vi "Event-Driven State Machine (Execution Log).vi"() -> ()   [LabVIEW 2020]
uses:
  support/States.ctl
  support/State Machine Data.ctl
  <vilib>/DAQmx/read.llb/DAQmx Read (Analog 2D DBL NChan NSamp).vi
  <vilib>/DAQmx/write.llb/DAQmx Write (Analog DBL 1Chan 1Samp).vi
  <vilib>/DAQmx/create/channels.llb/DAQmx Create Channel (AI-Voltage-Basic).vi
  <vilib>/DAQmx/configure/timing.llb/DAQmx Timing (Sample Clock).vi
  <vilib>/DAQmx/miscellaneous.llb/DAQmx Fill In Error Info.vi
  <vilib>/Utility/file.llb/Write Delimited Spreadsheet (DBL).vi
  <vilib>/DAQmx/create/channels.llb/DAQmx Create Channel (AO-Voltage-Basic).vi
panel:
  out "RMS Results Per Channel":dbl[](array[numeric])
  in  "AO Voltage Channel":tag="PCI-6221/ao1"
  in  "Generate Stimulus":bool
  out "Threshold exceeded?":bool
  in  "Acquire":bool
  in  "Samples per channel":i32=100
  in  "Sample Rate (Hz)":dbl=1000.0
  in  "AI Voltage Channel":tag="PCI-6221/ai0, PCI-6221/ai2:3"
  in  "Threshold (rms)":dbl=1.0
  in  "Clear":bool
  in  "Exit":bool
  out "Graph":dbl[][](graph)
  # "Analysis"
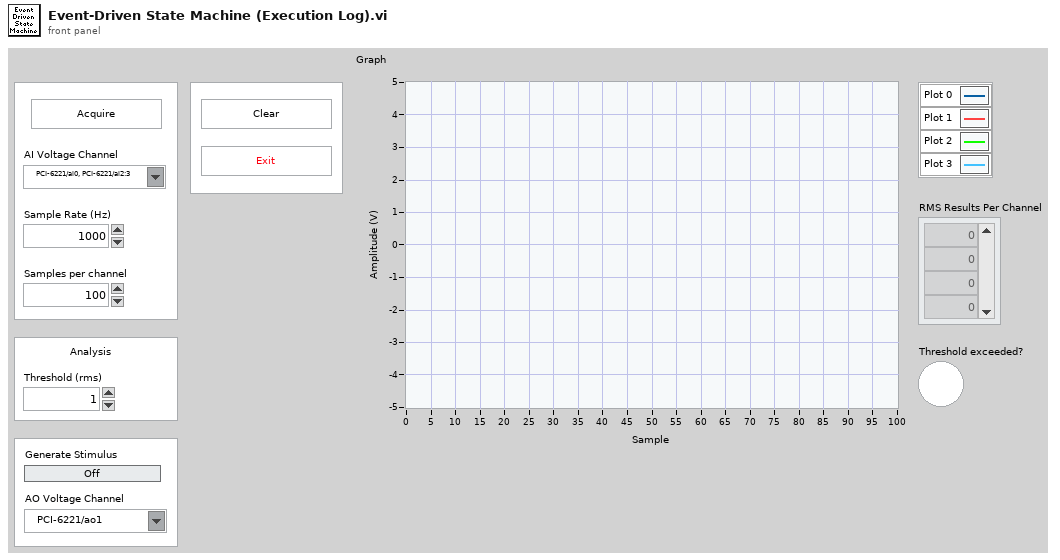
[diagram p1: front panel]
types:
  T1 = enum16{"open", "replace", "create", "open or create", "replace or create", "replace or create with confirmation"}
  T2 = typedef "State Machine Data.ctl" = cluster{"Acquisition Data":dbl[][], "Stimulus Value":bool}
  T3 = typedef "States.ctl" = enum16{"Initialize", "Wait for Event", "Acquire", "Analyze", "Log", "Clear", "Update UI", "Update Stumulus", "Exit"}
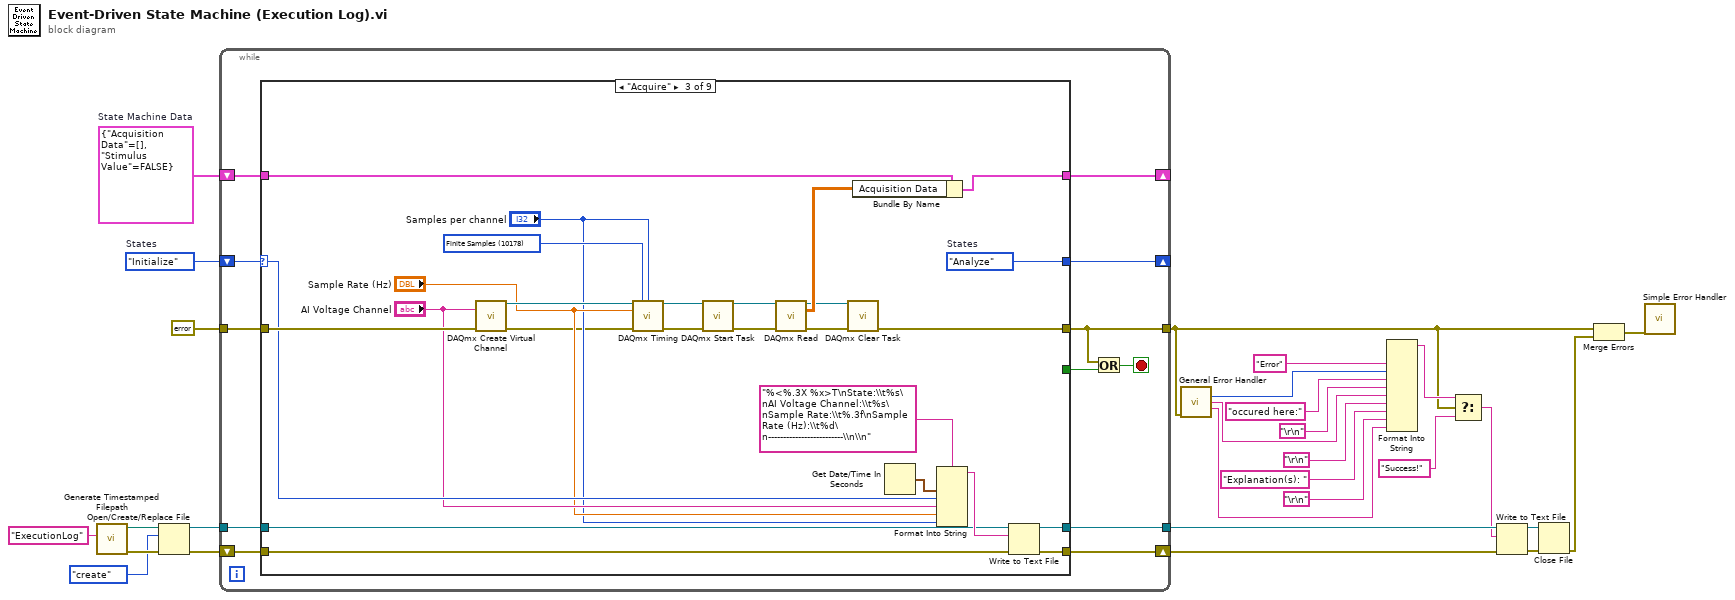
[diagram p0: block diagram]
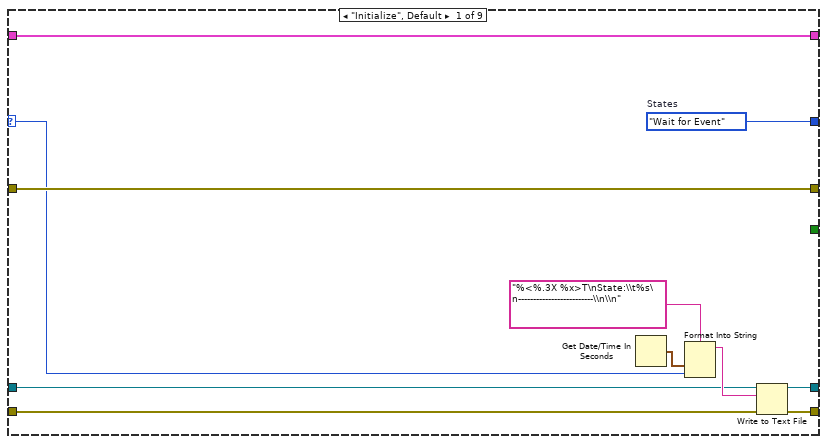
[diagram p2: hidden frame]
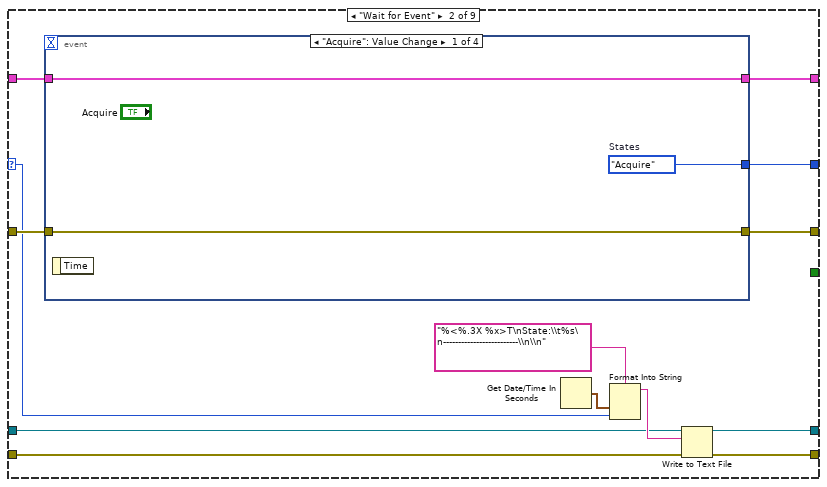
[diagram p3: hidden frame]
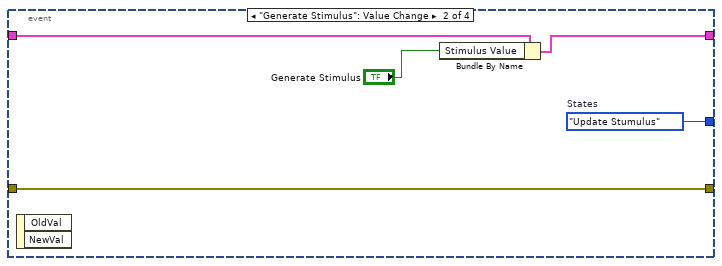
[diagram p4: hidden frame]
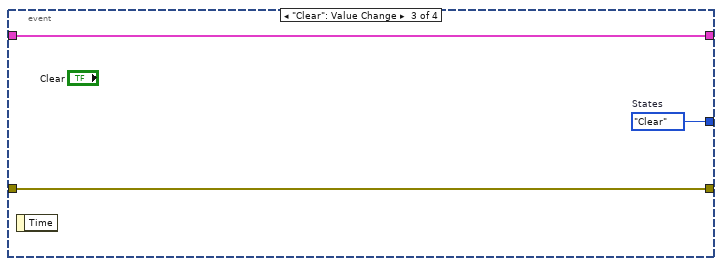
[diagram p5: hidden frame]
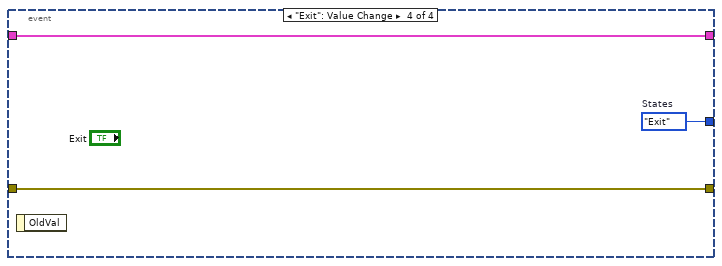
[diagram p6: hidden frame]
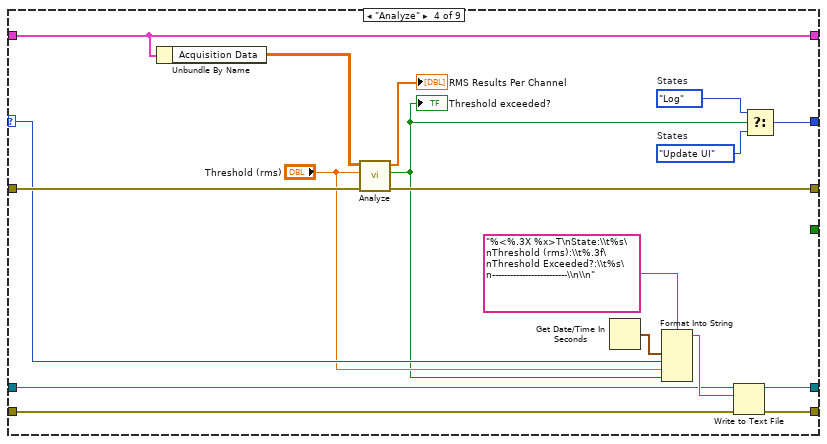
[diagram p7: hidden frame]
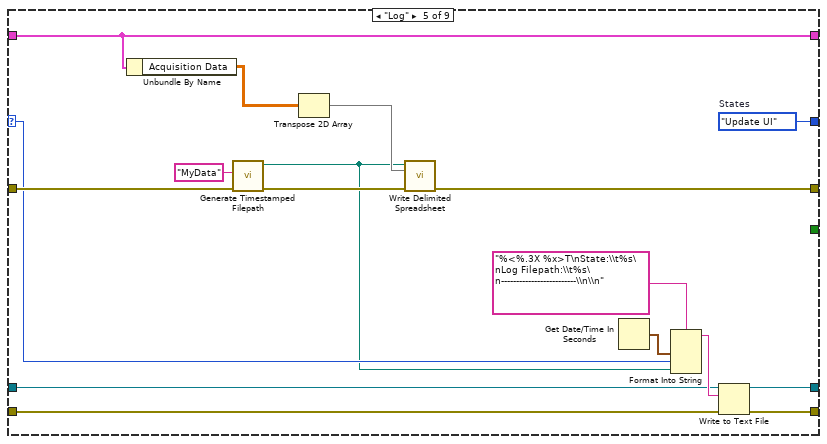
[diagram p8: hidden frame]
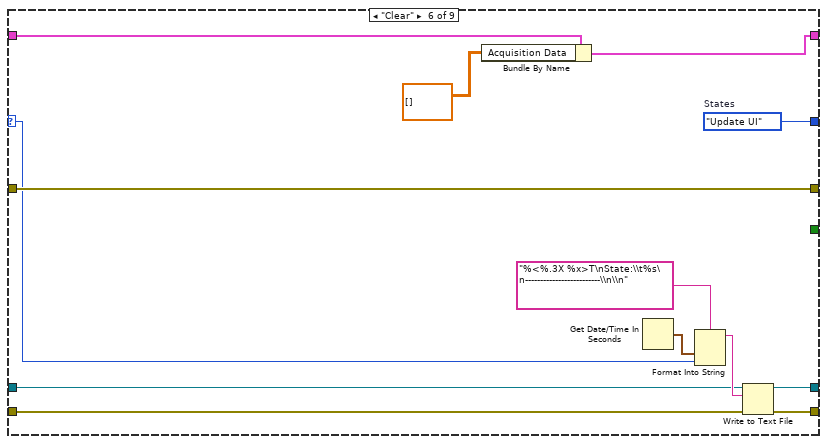
[diagram p9: hidden frame]
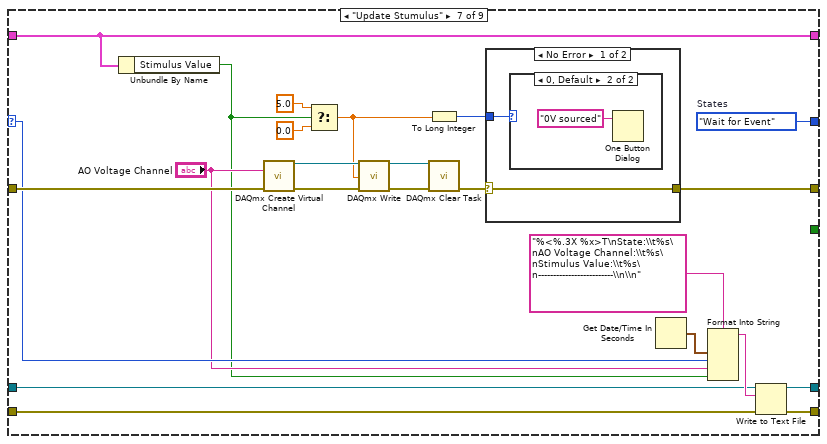
[diagram p10: hidden frame]
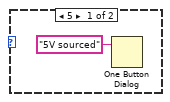
[diagram p11: hidden frame]
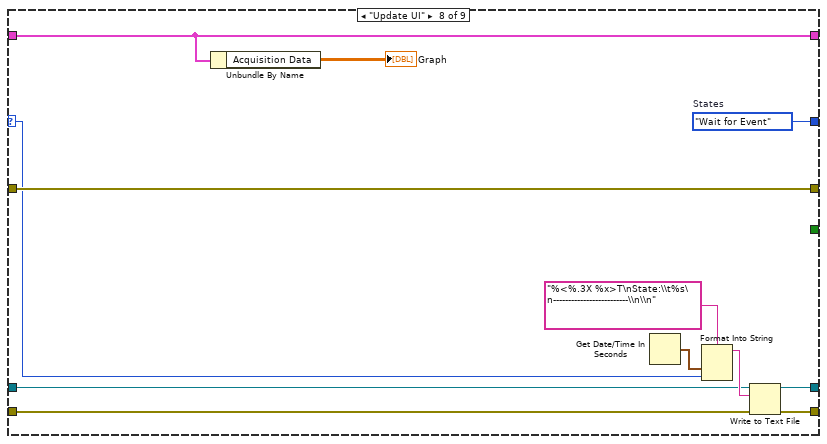
[diagram p13: hidden frame]
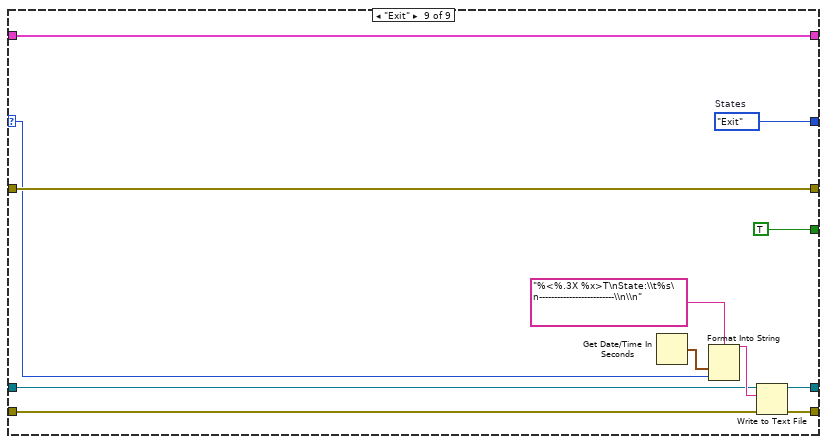
[diagram p14: hidden frame]
diagram:
  w28 = T2 {"Acquisition Data"=[], "Stimulus Value"=FALSE}  # State Machine Data
  w27 = States."Initialize"  # States
  n1 = call "Generate Timestamped Filepath.vi"("appended filename"="ExecutionLog") -> ("Error Out"=w24:errorcluster, "timestamped relative filepath"=w25:path)  [unwired: 9 in]
  n2 = Open/Create/Replace File(file path (use dialog)=w25, error in=w24, operation (0:open)=T1."create") -> (refnum out=w21:refnum<file>, error out=w20:errorcluster)  [unwired: 3 in, 1 out]
  n3 = while {
    tunnel: errorcluster {"status"=FALSE, "code"=0, "source"=""} ("error constant") -> [w39]
    tunnel: [w35] -> w2
    shift-right: [w37] -> _
    shift-left: w28 -> [w38]
    shift-right: [w36] -> _
    shift-left: w27 -> [w40]
    tunnel: w21 -> [w32]
    shift-right: [w30] -> w9
    shift-left: w20 -> [w31]
    tunnel: [w29] -> w10
    stop <- w34 stop-if-true
    n4 = case shown="\"Acquire\"" w40 {
      selector: w40 -> [w45 w52 w83 w108 w125 w141 w158 w182 w194]
      tunnel: w39 -> [w51 w62 w104 w121 w138 w152 w165 w191 w203]
      tunnel: [w51 w61 w100 w120 w133 w152 w156 w191 w203] -> w35
      tunnel: [w50 w63 w97 w122 w139 w150 w175 w192 w204] -> w37
      tunnel: w38 -> [w50 w64 w98 w122 w139 w151 w175 w192 w204]
      tunnel: [w49 w60 w99 w116 w132 w148 w166 w190 w201] -> w36
      tunnel: [_ _ _ _ _ _ _ _ TRUE] -> w33
      tunnel: w32 -> [w42 w54 w85 w110 w127 w143 w160 w184 w196]
      tunnel: w31 -> [w48 w57 w84 w109 w126 w142 w159 w183 w195]
      tunnel: [w47 w56 w86 w111 w128 w144 w161 w185 w197] -> w30
      tunnel: [w41 w55 w87 w112 w129 w145 w162 w186 w198] -> w29
      frame "Initialize", Default {
        w49 = States."Wait for Event"  # States
        n5 = Get Date/Time In Seconds() -> (seconds since 1Jan1904=w46:timestamp)
        n6 = Format Into String(format string="%<%.3X %x>T\nState:\\t%s\n-------------------------\\n\\n", w46, w45) -> (resulting string=w43:string)  [unwired: 2 in, 1 out]
        n7 = Write to Text File(file (use dialog)=w42, text=w43, error in=w48) -> (refnum out=w41:refnum<file>, error out=w47:errorcluster)  [unwired: 1 in, 1 out]
      }
      frame "Wait for Event" {
        n8 = event shown="[0] \"Acquire\": Value Change" {
          selector: _ -> [_ _ _ _]
          dyn-events: _ -> [_ _ _ _]
          timeout: _ -> [_ _ _ _]
          tunnel: w64 -> [w67 w72 w75 w77]
          tunnel: [w67 w71 w75 w77] -> w63
          tunnel: w62 -> [w66 w68 w74 w78]
          tunnel: [w66 w68 w74 w78] -> w61
          tunnel: [w65 w69 w73 w76] -> w60
          event "Acquire": Value Change {
            w65 = States."Acquire"  # States
            n9 = event-data() -> ()  [unwired: 1 in, 1 out]
          }
          event "Generate Stimulus": Value Change {
            w69 = States."Update Stumulus"  # States
            n10 = event-data() -> ()  [unwired: 1 in, 2 out]
            n11 = Bundle By Name(cluster=w72, "Stimulus Value"="Generate Stimulus") -> (w71:T2)
          }
          event "Clear": Value Change {
            w73 = States."Clear"  # States
            n12 = event-data() -> ()  [unwired: 1 in, 1 out]
          }
          event "Exit": Value Change {
            w76 = States."Exit"  # States
            n13 = event-data() -> ()  [unwired: 1 in, 1 out]
          }
        }
        n14 = Get Date/Time In Seconds() -> (seconds since 1Jan1904=w59:timestamp)
        n15 = Format Into String(format string="%<%.3X %x>T\nState:\\t%s\n-------------------------\\n\\n", w59, w52) -> (resulting string=w58:string)  [unwired: 2 in, 1 out]
        n16 = Write to Text File(file (use dialog)=w54, text=w58, error in=w57) -> (refnum out=w55:refnum<file>, error out=w56:errorcluster)  [unwired: 1 in, 1 out]
      }
      frame "Acquire" {
        w96 = 10178 items=["Finite Samples"=10178, "Continuous Samples"=10123, "Hardware Timed Single Point"=12522] ("sample mode")
        w99 = States."Analyze"  # States
        n17 = call-poly <vilib>:"DAQmx Create Virtual Channel.vi"("physical channels"="AI Voltage Channel", "error in"=w104) -> ("task out"=w94:refnum<k21>, "error out"=w79:errorcluster)  [unwired: 12 in]
        n18 = call-poly <vilib>:"DAQmx Timing.vi"("task/channels in"=w94, "sample mode"=w96, "samples per channel"="Samples per channel", "rate"="Sample Rate (Hz)", "error in"=w79) -> ("task out"=w93:refnum<k21>, "error out"=w103:errorcluster)  [unwired: 9 in]
        n19 = call <vilib>:"DAQmx Start Task.vi"("task/channels in"=w93, "error in"=w103) -> ("task out"=w92:refnum<k21>, "error out"=w102:errorcluster)  [unwired: 12 in]
        n20 = call-poly <vilib>:"DAQmx Read.vi"("task/channels in"=w92, "error in"=w102) -> ("task out"=w91:refnum<k21>, "data"=w95:dbl[][], "error out"=w101:errorcluster)  [unwired: 11 in]
        n21 = call <vilib>:"DAQmx Clear Task.vi"("task in"=w91, "error in"=w101) -> ("error out"=w100:errorcluster)  [unwired: 13 in]
        n22 = Bundle By Name(cluster=w98, "Acquisition Data"=w95) -> (w97:T2)
        n23 = Get Date/Time In Seconds() -> (seconds since 1Jan1904=w89:timestamp)
        n24 = Format Into String(format string="%<%.3X %x>T\nState:\\t%s\nAI Voltage Channel:\\t%s\nSample Rate:\\t%.3f\nSample Rate (Hz):\\t%d\n-------------------------\\n\\n", w89, w83, "AI Voltage Channel", "Sample Rate (Hz)", "Samples per channel") -> (resulting string=w90:string)  [unwired: 2 in, 1 out]
        n25 = Write to Text File(file (use dialog)=w85, text=w90, error in=w84) -> (refnum out=w87:refnum<file>, error out=w86:errorcluster)  [unwired: 1 in, 1 out]
      }
      frame "Analyze" {
        w117 = States."Update UI"  # States
        w118 = States."Log"  # States
        n26 = Unbundle By Name(w122) -> ("Acquisition Data"=w119:dbl[][])
        n27 = call "Analyze.vi"("Error In"=w121, "Treshold (rms)"="Threshold (rms)", "N-Channel Data (2D DBL)"=w119) -> ("Error Out"=w120:errorcluster, "Threshold exceeded?"=w106:bool, "N-Channel Data RMS Results"=→"RMS Results Per Channel":dbl[])  [unwired: 5 in, 1 out]
        "Threshold exceeded?" <- w106
        n28 = Get Date/Time In Seconds() -> (seconds since 1Jan1904=w114:timestamp)
        n29 = Format Into String(format string="%<%.3X %x>T\nState:\\t%s\nThreshold (rms):\\t%.3f\nThreshold Exceeded?:\\t%s\n-------------------------\\n\\n", w114, w108, "Threshold (rms)", w106) -> (resulting string=w113:string)  [unwired: 2 in, 1 out]
        n30 = Write to Text File(file (use dialog)=w110, text=w113, error in=w109) -> (refnum out=w112:refnum<file>, error out=w111:errorcluster)  [unwired: 1 in, 1 out]
        n31 = Select(t=w118, s=w106, f=w117) -> (s? t:f=w116:T3)
      }
      frame "Log" {
        w132 = States."Update UI"  # States
        n32 = Unbundle By Name(w139) -> ("Acquisition Data"=w136:dbl[][])
        n33 = call "Generate Timestamped Filepath.vi"("Error In"=w138, "appended filename"="MyData") -> ("Error Out"=w134:errorcluster, "timestamped relative filepath"=w124:path)  [unwired: 8 in]
        n34 = Transpose 2D Array(2D array=w136) -> (transposed array=w135:dbl[][])
        n35 = call-poly <vilib>:"Write Delimited Spreadsheet.vi"("file path (dialog if empty)"=w124, "2D data"=w135, "error in (no error)"=w134) -> ("error out"=w133:errorcluster)  [unwired: 11 in, 1 out]
        n36 = Get Date/Time In Seconds() -> (seconds since 1Jan1904=w131:timestamp)
        n37 = Format Into String(format string="%<%.3X %x>T\nState:\\t%s\nLog Filepath:\\t%s\n-------------------------\\n\\n", w131, w125, w124) -> (resulting string=w130:string)  [unwired: 2 in, 1 out]
        n38 = Write to Text File(file (use dialog)=w127, text=w130, error in=w126) -> (refnum out=w129:refnum<file>, error out=w128:errorcluster)  [unwired: 1 in, 1 out]
      }
      frame "Clear" {
        w148 = States."Update UI"  # States
        n39 = Bundle By Name(cluster=w151, "Acquisition Data"=dbl[][] []) -> (w150:T2)
        n40 = Get Date/Time In Seconds() -> (seconds since 1Jan1904=w146:timestamp)
        n41 = Format Into String(format string="%<%.3X %x>T\nState:\\t%s\n-------------------------\\n\\n", w146, w141) -> (resulting string=w147:string)  [unwired: 2 in, 1 out]
        n42 = Write to Text File(file (use dialog)=w143, text=w147, error in=w142) -> (refnum out=w145:refnum<file>, error out=w144:errorcluster)  [unwired: 1 in, 1 out]
      }
      frame "Update Stumulus" {
        w166 = States."Wait for Event"  # States
        n43 = Unbundle By Name(w175) -> ("Stimulus Value"=w154:bool)
        n44 = call-poly <vilib>:"DAQmx Create Virtual Channel.vi"("physical channels"="AO Voltage Channel", "error in"=w165) -> ("task out"=w172:refnum<k21>, "error out"=w171:errorcluster)  [unwired: 12 in]
        n45 = Select(t=5.0, s=w154, f=0.0) -> (s? t:f=w168:dbl)
        n46 = call-poly <vilib>:"DAQmx Write.vi"("task/channels in"=w172, "data"=w168, "error in"=w171) -> ("task out"=w170:refnum<k21>, "error out"=w169:errorcluster)  [unwired: 10 in, 1 out]
        n47 = To Long Integer(number=w168) -> (32bit integer=w167:i32)
        n48 = call <vilib>:"DAQmx Clear Task.vi"("task in"=w170, "error in"=w169) -> ("error out"=w157:errorcluster)  [unwired: 13 in]
        n49 = case shown="No Error" w157 {
          selector: w157 -> [w176 w180]
          tunnel: w167 -> [w177 _]
          tunnel: [w176 w180] -> w156
          frame No Error {
            n50 = case shown="0, Default" w177 {
              frame 5 {
                n51 = One Button Dialog(message="5V sourced") -> ()  [unwired: 1 in, 1 out]
              }
              frame 0, Default {
                n52 = One Button Dialog(message="0V sourced") -> ()  [unwired: 1 in, 1 out]
              }
            }
          }
          frame Error {
          }
        }
        n53 = Get Date/Time In Seconds() -> (seconds since 1Jan1904=w164:timestamp)
        n54 = Format Into String(format string="%<%.3X %x>T\nState:\\t%s\nAO Voltage Channel:\\t%s\nStimulus Value:\\t%s\n-------------------------\\n\\n", w164, w158, "AO Voltage Channel", w154) -> (resulting string=w163:string)  [unwired: 2 in, 1 out]
        n55 = Write to Text File(file (use dialog)=w160, text=w163, error in=w159) -> (refnum out=w162:refnum<file>, error out=w161:errorcluster)  [unwired: 1 in, 1 out]
      }
      frame "Update UI" {
        w190 = States."Wait for Event"  # States
        n56 = Unbundle By Name(w192) -> ("Acquisition Data"=→"Graph":dbl[][])
        n57 = Get Date/Time In Seconds() -> (seconds since 1Jan1904=w187:timestamp)
        n58 = Format Into String(format string="%<%.3X %x>T\nState:\\t%s\n-------------------------\\n\\n" ("initial string"), w187, w182) -> (resulting string=w188:string)  [unwired: 2 in, 1 out]
        n59 = Write to Text File(file (use dialog)=w184, text=w188, error in=w183) -> (refnum out=w186:refnum<file>, error out=w185:errorcluster)  [unwired: 1 in, 1 out]
      }
      frame "Exit" {
        w201 = States."Exit"  # States
        n60 = Get Date/Time In Seconds() -> (seconds since 1Jan1904=w200:timestamp)
        n61 = Format Into String(format string="%<%.3X %x>T\nState:\\t%s\n-------------------------\\n\\n", w200, w194) -> (resulting string=w199:string)  [unwired: 2 in, 1 out]
        n62 = Write to Text File(file (use dialog)=w196, text=w199, error in=w195) -> (refnum out=w198:refnum<file>, error out=w197:errorcluster)  [unwired: 1 in, 1 out]
      }
    }
    n63 = Or(x=w35, y=w33) -> (x .or. y?=w34:bool)
  }
  n64 = call <vilib>:"General Error Handler.vi"("error in (no error)"=w2) -> ("code out"=w13:i32, "source out"=w12:string, "message"=w11:string)  [unwired: 10 in, 2 out]
  n65 = Format Into String("Error", w13, "occured here:" ("input 3"), "\r\n", w12, "\r\n", "Explanation(s): ", "\r\n", w11) -> (resulting string=w8:string)  [unwired: 3 in, 1 out]
  n66 = Select(t=w8, s=w2, f="Success!") -> (s? t:f=w6:string)
  n67 = Write to Text File(file (use dialog)=w10, text=w6, error in=w9) -> (refnum out=w5:refnum<file>, error out=w4:errorcluster)  [unwired: 1 in, 1 out]
  n68 = Close File(refnum=w5, error in=w4) -> (error out=w3:errorcluster)  [unwired: 1 out]
  n69 = Merge Errors(w2, w3) -> (w1:errorcluster)
  n70 = call <vilib>:"Simple Error Handler.vi"("error in (no error)"=w1) -> ()  [unwired: 4 in, 5 out]
